vi "Calibration (SubVI).vi"(8 "error constant":errorcluster) -> (0 "error constant 2":errorcluster, 1 "Val":dbl[](array[numeric]), 2 "K":u32[](array[numeric]))   [LabVIEW 2017]
panel:
  in  "OK Button":bool
  in  "Boolean 14":bool
  in  "Boolean 13":bool
  in  "Boolean 12":bool
  in  "Boolean 11":bool
  in  "Boolean 10":bool
  in  "Boolean 9":bool
  in  "Boolean 8":bool
  in  "Boolean 7":bool
  in  "Boolean 6":bool
  in  "Boolean 5":bool
  in  "Boolean 4":bool
  in  "Boolean 3":bool
  in  "Boolean 2":bool
  in  "Boolean":bool
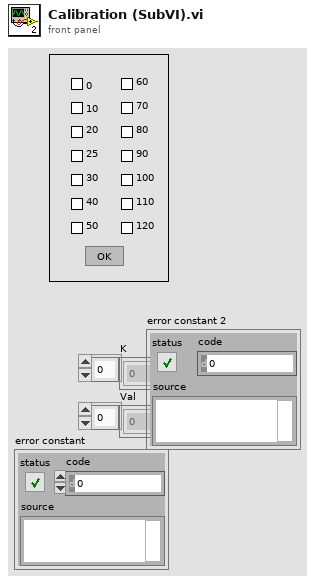
[diagram p1: front panel]
types:
  T1 = enum32{"Invalid", "Standard", "Closed", "Hidden", "Minimized", "Maximized"}
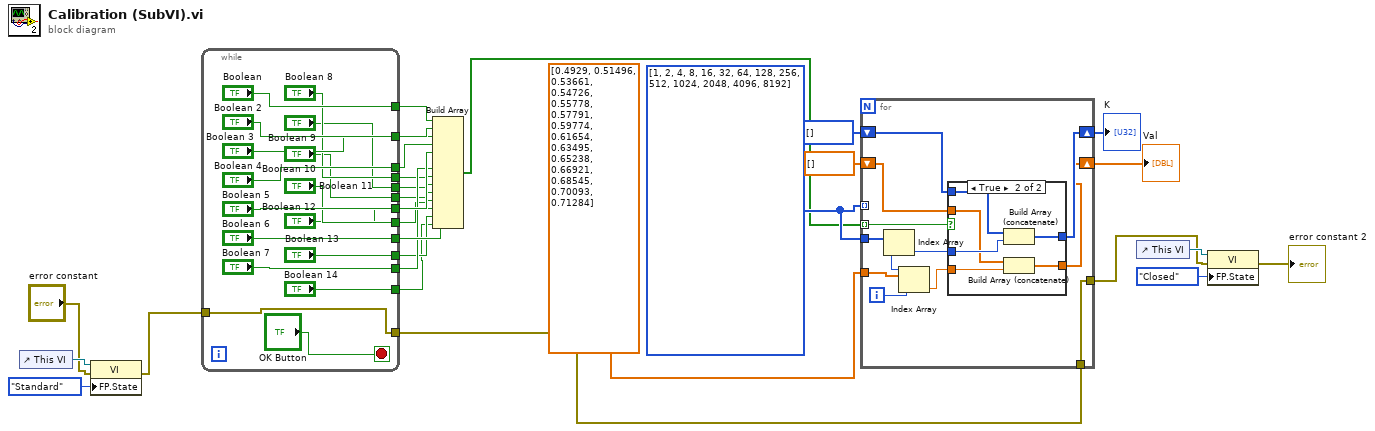
[diagram p0: block diagram]
diagram:
  w30 = u32[] [1, 2, 4, 8, 16, 32, 64, 128, 256, 512, 1024, 2048, 4096, 8192] ("appended array")
  n1 = control-ref of="This VI"() -> (w5:refnum<vi>)
  n2 = property class="VI"(reference=w5, error in="error constant", "FP.State"=T1."Standard" ("Front Panel Window:State")) -> (error out=w1:errorcluster)  [unwired: 1 out]
  n3 = while {
    tunnel: ["Boolean"] -> w26
    tunnel: ["Boolean 2"] -> w25
    tunnel: ["Boolean 3"] -> w24
    tunnel: ["Boolean 4"] -> w23
    tunnel: ["Boolean 5"] -> w22
    tunnel: ["Boolean 6"] -> w21
    tunnel: ["Boolean 7"] -> w20
    tunnel: ["Boolean 8"] -> w19
    tunnel: ["Boolean 9"] -> w18
    tunnel: ["Boolean 10"] -> w17
    tunnel: ["Boolean 11"] -> w16
    tunnel: ["Boolean 12"] -> w15
    tunnel: ["Boolean 13"] -> w14
    tunnel: ["Boolean 14"] -> w13
    tunnel: [w31] -> w3
    tunnel: w1 -> [w31]
    stop <- "OK Button" stop-if-true
  }
  n4 = Build Array(w26, w25, w24, w23, w22, w21, w20, w19, w18, w17, w16, w15, w14, w13) -> (w12:bool[])
  n5 = for {
    tunnel: w30 -> [_] mode=indexing
    tunnel: w30 -> [w57]
    tunnel: dbl[] [0.4929, 0.51496, 0.53661, 0.54726, 0.55778, 0.57791, 0.59774, 0.61654, 0.63495, 0.65238, 0.66921, 0.68545, 0.70093, 0.71284] -> [w56]
    shift-right: [w50] -> w11
    shift-left: u32[] [] -> [w52]
    shift-right: [w49] -> w10
    shift-left: dbl[] [] -> [w51]
    tunnel: w12 -> [w48] mode=indexing
    tunnel: [w47] -> w7
    tunnel: w3 -> [w47]
    i -> [w55]
    n6 = Index Array(array=w57, index=w55) -> (element=w53:u32)
    n7 = Index Array(array=w56, index=w55) -> (element=w54:dbl)
    n8 = case shown="True" w48 {
      tunnel: w54 -> [_ w61]
      tunnel: w53 -> [_ w64]
      tunnel: w52 -> [w59 w65]
      tunnel: w51 -> [w58 w62]
      tunnel: [w59 w63] -> w50
      tunnel: [w58 w60] -> w49
      frame False {
      }
      frame True {
        n9 = Build Array (concatenate)(w65, w64) -> (w63:u32[])
        n10 = Build Array (concatenate)(w62, w61) -> (w60:dbl[])
      }
    }
  }
  "K" <- w11
  "Val" <- w10
  n11 = control-ref of="This VI"() -> (w9:refnum<vi>)
  n12 = property class="VI"(reference=w9, error in=w7, "FP.State"=T1."Closed" ("Front Panel Window:State")) -> (error out=→"error constant 2":errorcluster)  [unwired: 1 out]
